vi "Network Stream Transmitter.vi"() -> ()   [LabVIEW 2020]
uses:
  Type Definitions/Payload Class.ctl
  Type Definitions/Data Frame Header.ctl
  Type Definitions/Data Frame.ctl
  <vilib>/dex/Stream Element Allocation Mode.ctl
  <resource>/objmgr/ni.dex.rc
  Type Definitions/Telemetry TCP State.ctl
  <vilib>/platform/TimedLoop/XDataNode/XDataNode.xnode
  <vilib>/Platform/TimedLoop/XDataNode/nitl_modes.ctl
  <vilib>/Platform/TimedLoop/XDataNode/XDNodeRunTimeDep.lvlib
  <vilib>/Platform/TimedLoop/XDataNode/wakeup.ctl
  <vilib>/Platform/TimedLoop/XDataNode/timing_clust.ctl
  Type Definitions/Enum - System State.ctl
panel:
  out "Network Stream Status":T1
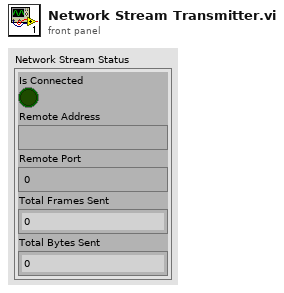
[diagram p1: front panel]
types:
  T1 = typedef "Telemetry TCP State.ctl" = cluster{"Is Connected":bool, "Remote Address":string, "Remote Port":u16, "Total Frames Sent":i32, "Total Bytes Sent":i32}
  T2 = typedef "XDNodeRunTimeDep.lvlib/timing_clust.ctl" = cluster{"Expected End [f-1]":u64, "Actual End [f-1]":u64, "Finished Late? [f-1]":bool, "Expected End [i-1]":u64, "Actual End [i-1]":u64, "Finished Late? [i-1]":bool, "Expected Start [i]":u64, "Actual Start [i]":u64, "Expected Start [f]":u64, "Actual Start [f]":u64, "Source Name":string, "Structure Name":string, "Period":i64, "Deadline":i64, "Offset":i64, "Start":i64, "Priority":i32, "Timeout":i32, "Mode":T3, "Wakeup Reason":T4, "Error":errorcluster, "Source Type":string, "Secondary Source Type":string, "Global End Time":u64, "Global Start Time":u64, "Frame Duration":u64, "Iteration Duration":u64, "Assigned CPU":i32, "I/O Scan Engine Mode":u32}
  T3 = typedef "XDNodeRunTimeDep.lvlib/nitl_modes.ctl" = enum32{"No Change", "Process missed periods, maintain original phase", "Discard missed periods, maintain original phase", "Process missed periods, ignore original phase", "Discard missed periods, ignore original phase"}
  T4 = typedef "XDNodeRunTimeDep.lvlib/wakeup.ctl" = enum32{"Normal", "Aborted", "Asynchronous wakeup", "Timing source error", "Timed loop error", "Timeout"}
  T5 = typedef "Data Frame.ctl" = cluster{"Frame Header":T6, "Payload":string, "CRC":u32}
  T6 = typedef "Data Frame Header.ctl" = cluster{"Sync":u32, "Time":dbl, "Microsecond Clock":u64, "Payload Class":T7, "Payload ID":u16, "Counter":u32, "Options":u32, "Source":i32, "Destination":i32}
  T7 = typedef "Payload Class.ctl" = enum16{"System State", "Parameters", "Metadata", "Software Monitor", "Data", "Commands"}
  T8 = typedef "Enum - System State.ctl" = enum16{"System Time", "Telemetry Network Stream Status", "Writeable Drives", "Command Network Stream Status", "Network Adapters", "UDP Discovery Engine Metadata"}
  T9 = typedef "Stream Element Allocation Mode.ctl" = u32
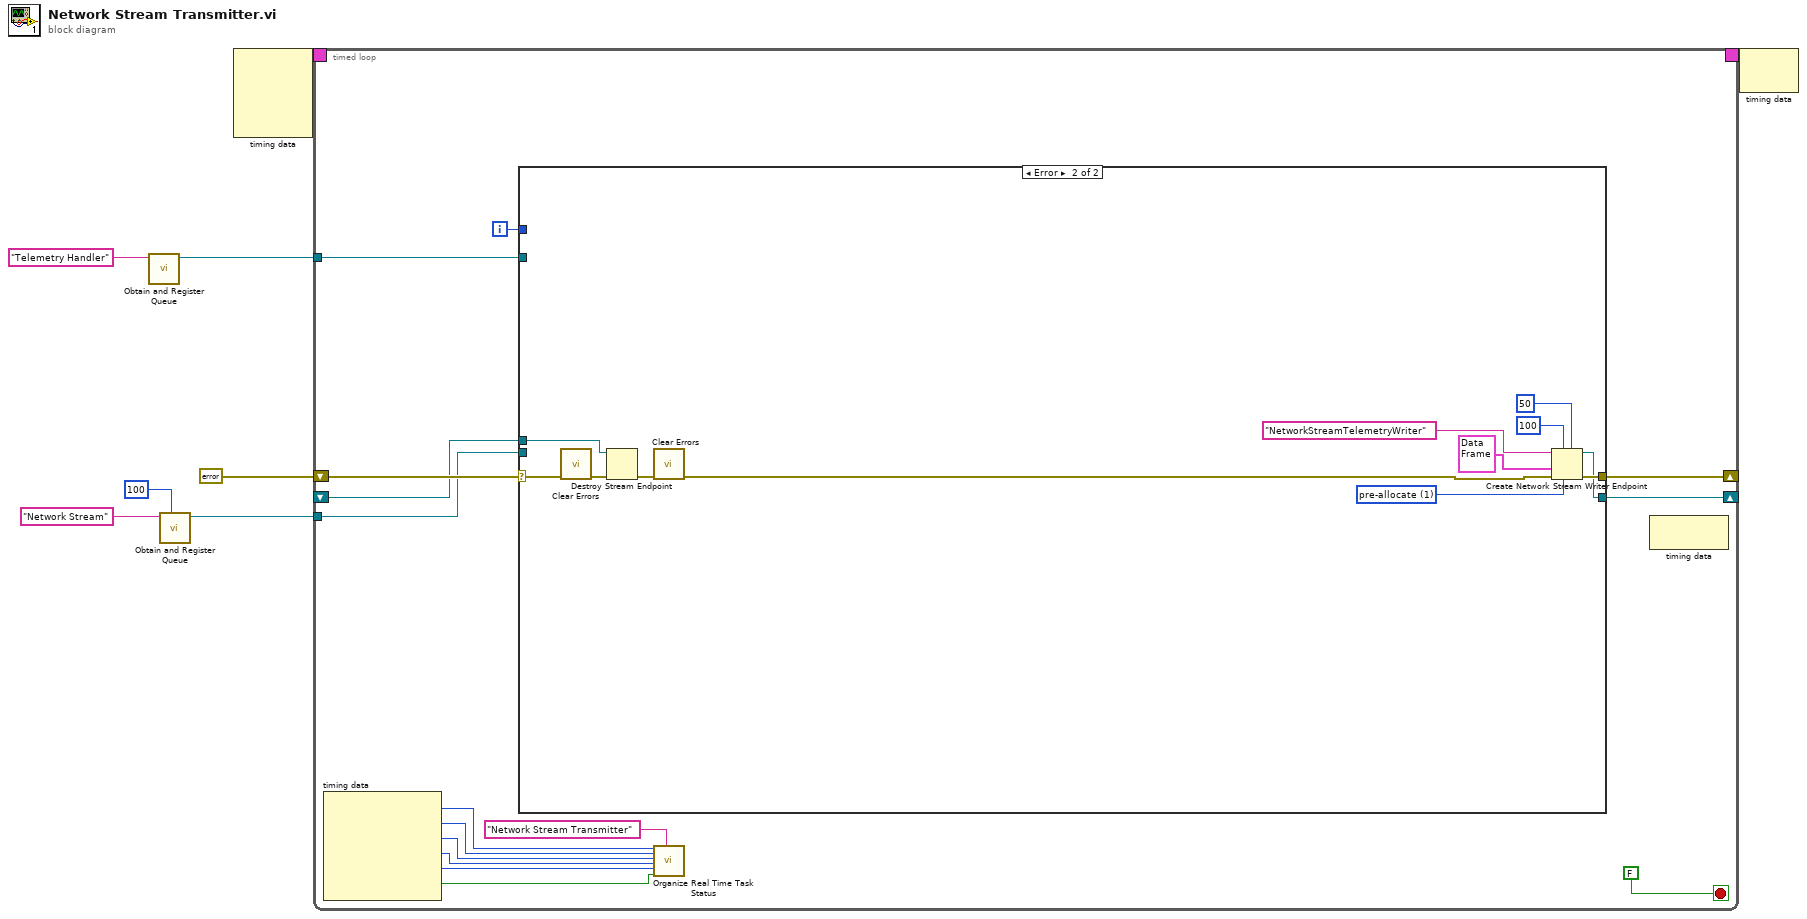
[diagram p0: block diagram]
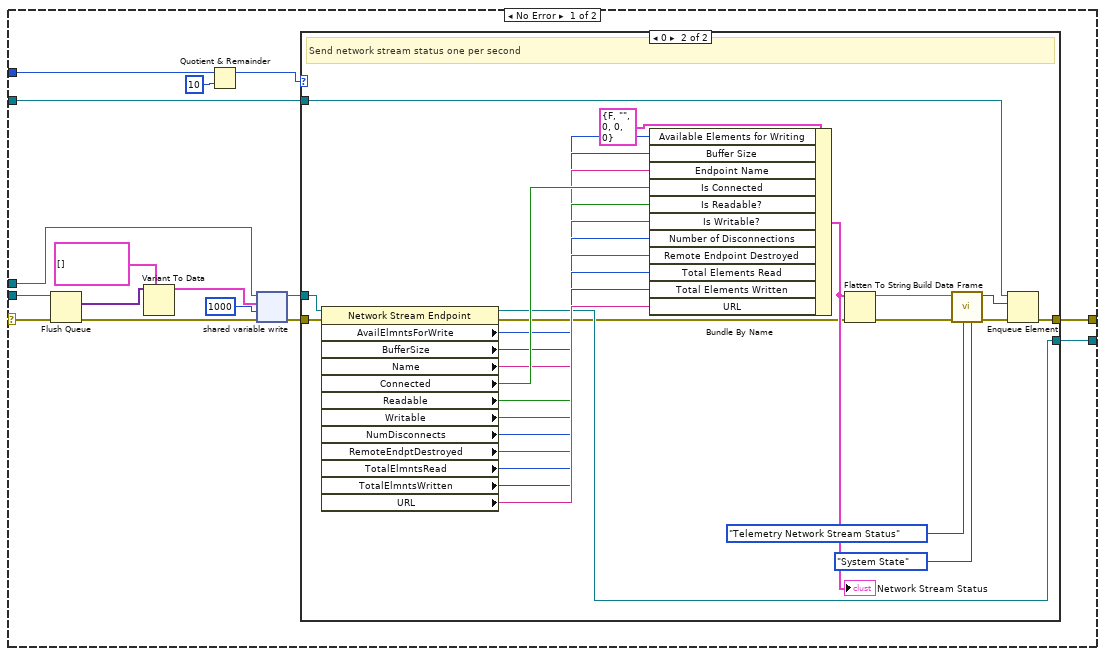
[diagram p2: hidden frame]
diagram:
  n1 = call "Obtain and Register Queue.vi"("name (unnamed)"="Telemetry Handler") -> ("Queue Out"=w1:refnum<queue>)  [unwired: 7 in, 3 out]
  n2 = call "Obtain and Register Queue.vi"("max queue size (-1, unlimited)"=100, "name (unnamed)"="Network Stream") -> ("Queue Out"=w5:refnum<queue>)  [unwired: 6 in, 3 out]
  n3 = node-c288() -> (w3:T2)  [unwired: 4 in]
  n4 = timed-loop {
    shift-right: [w17] -> _
    shift-left: errorcluster {"status"=TRUE, "code"=0, "source"=""} ("error out") -> [w23]
    shift-right: [w18] -> _
    shift-left: _ -> [w20]
    tunnel: w5 -> [w22]
    timing: w3 -> [_]
    timing-out: [_] -> w2
    tunnel: w1 -> [w19]
    i -> [w16]
    stop <- FALSE stop-if-true
    n5 = node-c288() -> (w14:i32, w13:i32, w12:i64, w11:i64, w10:i64, w9:bool)  [unwired: 1 in]
    n6 = case shown="Error" w23 {
      selector: w23 -> [w46 w80]
      tunnel: [w36 w85] -> w17
      tunnel: [w38 w84] -> w18
      tunnel: w20 -> [w44 w82]
      tunnel: w22 -> [w47 _]
      tunnel: w19 -> [w40 _]
      tunnel: w16 -> [w35 _]
      frame No Error {
        n7 = Flush Queue(queue=w47, error in (no error)=w46) -> (remaining elements=w45:variant[], error out=w43:errorcluster)  [unwired: 1 out]
        n8 = Variant To Data(type=T5[] [] ("Array"), Variant=w45) -> (data=w42:T5[])  [unwired: 1 in, 1 out]
        n9 = Quotient & Remainder(x=w35, y=10) -> (x-y*floor(x/y)=w33:i32)  [unwired: 1 out]
        n10 = shared-variable-write(w44, w43, w42, 1000 ("timeout ms (-1)")) -> (w39:refnum<k21>, w37:errorcluster)  [unwired: 1 out]
        n11 = case shown="0" w33 {
          tunnel: w40 -> [_ w57]
          tunnel: w39 -> [w49 w56]
          tunnel: [w49 w55] -> w38
          tunnel: w37 -> [w48 w54]
          tunnel: [w48 w50] -> w36
          frame Default {
            # "Don't Send Network Stream Status"
          }
          frame 0 {
            # "Send network stream status one per second"
            n12 = property class="Network Stream Endpoint"(reference=w56, error in=w54) -> (reference out=w55:refnum<k21>, error out=w53:errorcluster, "AvailElmntsForWrite"=w59:i32, "BufferSize"=w60:i32, "Name"=w61:string, "Connected"=w62:bool, "Readable"=w63:bool, "Writable"=w64:bool, "NumDisconnects"=w65:u32, "RemoteEndptDestroyed"=w66:bool, "TotalElmntsRead"=w67:u64, "TotalElmntsWritten"=w68:u64, "URL"=w69:string)
            n13 = Bundle By Name(cluster=T1 {"Is Connected"=FALSE, "Remote Address"="", "Remote Port"=0, "Total Frames Sent"=0, "Total Bytes Sent"=0} ("Network Stream Status"), "Available Elements for Writing"=w59, "Buffer Size"=w60, "Endpoint Name"=w61, "Is Connected"=w62, "Is Readable?"=w63, "Is Writable?"=w64, "Number of Disconnections"=w65, "Remote Endpoint Destroyed"=w66, "Total Elements Read"=w67, "Total Elements Written"=w68, "URL"=w69) -> (w74:T1)
            "Network Stream Status" <- w74
            n14 = Flatten To String(anything=w74, error in (no error)=w53) -> (data string=w72:string, error out=w52:errorcluster)  [unwired: 2 in, 1 out]
            n15 = call "Build Data Frame.vi"("Payload Class (Data)"=Payload_Class."System State", "Payload ID (0)"=Enum_-_System_State."Telemetry Network Stream Status" ("System State"), "error in (no error)"=w52, "Payload (Empty String)"=w72) -> ("error out"=w51:errorcluster, "Frame"=w71:variant)  [unwired: 6 in]
            n16 = Enqueue Element(queue=w57, element=w71, error in (no error)=w51) -> (error out=w50:errorcluster)  [unwired: 1 in, 2 out]
          }
        }
      }
      frame Error {
        w79 = T9 1 items=["allocate as needed", "pre-allocate"] ("element allocation mode")
        n17 = call <vilib>:"Clear Errors.vi"("error in (no error)"=w80) -> ("error out"=w83:errorcluster)  [unwired: 5 in, 1 out]
        n18 = Destroy Stream Endpoint(8:w83, 11:w82) -> (0:w81:errorcluster)
        n19 = call <vilib>:"Clear Errors.vi"("error in (no error)"=w81) -> ("error out"=w86:errorcluster)  [unwired: 5 in, 1 out]
        n20 = Create Network Stream Writer Endpoint(5:50 ("timeout in ms (-1)"), 6:w79, 7:100 ("writer buffer size"), 8:w86, 9:T5 {"Frame Header"={"Sync"=0, "Time"=0.0, "Microsecond Clock"=0, "Payload Class"=enum."System State", "Payload ID"=0, "Counter"=0, "Options"=0, "Source"=0, "Destination"=0}, "Payload"="", "CRC"=0} ("Frame"), 11:"NetworkStreamTelemetryWriter" ("writer name")) -> (0:w85:errorcluster, 3:w84:refnum<k21>)  [unwired: 1 in]
      }
    }
    n21 = call "Organize Real Time Task Status.vi"("Priority"=w14, "Processor"=w13, "Offset"=w12, "Iteration Duration"=w11, "Period"=w10, "Finished Late? [i-1]"=w9, "Task Name"="Network Stream Transmitter") -> ()  [unwired: 12 in, 1 out]
    n22 = node-c288() -> ()  [unwired: 1 in, 1 out]
  }
  n23 = node-c288(w2) -> ()  [unwired: 1 out]
